vi "SeCrTs-AI SEQ MAIN.vi"(8 "error IO":errorcluster, 11 "Message Queue":refnum<queue>) -> (0 "error Out":errorcluster)   [LabVIEW 2022 SP3]
uses:
  <vilib>/Platform/TimedLoop/XDataNode/timing_clust.ctl
  <vilib>/Platform/TimedLoop/XDataNode/nitl_modes.ctl
  <vilib>/Platform/TimedLoop/XDataNode/wakeup.ctl
  RT Controls/SeCrTs-FGV Read write.ctl
  <vilib>/platform/TimedLoop/XDataNode/XDataNode.xnode
  <vilib>/Platform/TimedLoop/XDataNode/XDNodeRunTimeDep.lvlib
panel:
  out "array":string[](array[string])
  out "result":bool
  out "output array":string[](array[string])
  out "Failure case Seq":string[](array[string])
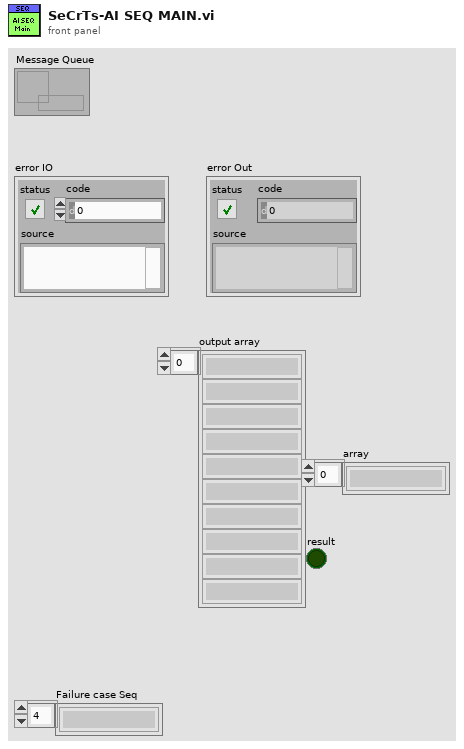
[diagram p1: front panel]
types:
  T1 = typedef "XDNodeRunTimeDep.lvlib/timing_clust.ctl" = cluster{"Expected End [f-1]":u64, "Actual End [f-1]":u64, "Finished Late? [f-1]":bool, "Expected End [i-1]":u64, "Actual End [i-1]":u64, "Finished Late? [i-1]":bool, "Expected Start [i]":u64, "Actual Start [i]":u64, "Expected Start [f]":u64, "Actual Start [f]":u64, "Source Name":string, "Structure Name":string, "Period":i64, "Deadline":i64, "Offset":i64, "Start":i64, "Priority":i32, "Timeout":i32, "Mode":T2, "Wakeup Reason":T3, "Error":errorcluster, "Source Type":string, "Secondary Source Type":string, "Global End Time":u64, "Global Start Time":u64, "Frame Duration":u64, "Iteration Duration":u64, "Assigned CPU":i32, "I/O Scan Engine Mode":u32}
  T2 = typedef "XDNodeRunTimeDep.lvlib/nitl_modes.ctl" = enum32{"No Change", "Process missed periods, maintain original phase", "Discard missed periods, maintain original phase", "Process missed periods, ignore original phase", "Discard missed periods, ignore original phase"}
  T3 = typedef "XDNodeRunTimeDep.lvlib/wakeup.ctl" = enum32{"Normal", "Aborted", "Asynchronous wakeup", "Timing source error", "Timed loop error", "Timeout"}
  T4 = typedef "SeCrTs-FGV Read write.ctl" = enum16{"Write", "Read"}
  T5 = cluster{"Manual HOLD":bool, "Automatic Hold AI":bool, "Abort":bool, "Automatic Hold DI":bool}
  T6 = cluster{"Start DAQ":bool, "Stop DAQ":bool, "RT Stop":bool, "RT Exit":bool, "Start Seq":bool}
  T7 = cluster{cluster{"Sr. No.":string, "Time CDT":string, "Component ID":string, "Data Type":string, "Condition":string, "Range/Position":string, "No of Samples for Pass":string, "Event Duration":string, "Continuous /Cumulative":string, "Expected Delay":string, "Failure case Seq":string, "Current Sequence":string}[]}[]
  T8 = cluster{"Sr. No.":string, "Time CDT":string, "Component ID":string, "Data Type":string, "Condition":string, "Range/Position":string, "No of Samples for Pass":string, "Event Duration":string, "Continuous /Cumulative":string, "Expected Delay":string, "Failure case Seq":string, "Current Sequence":string}[]
  T9 = cluster{"Sr. No.":string, "Time CDT":string, "Component ID":string, "Data Type":string, "Condition":string, "Range/Position":string, "No of Samples for Pass":string, "Event Duration":string, "Continuous /Cumulative":string, "Expected Delay":string, "Failure case Seq":string, "Current Sequence":string}
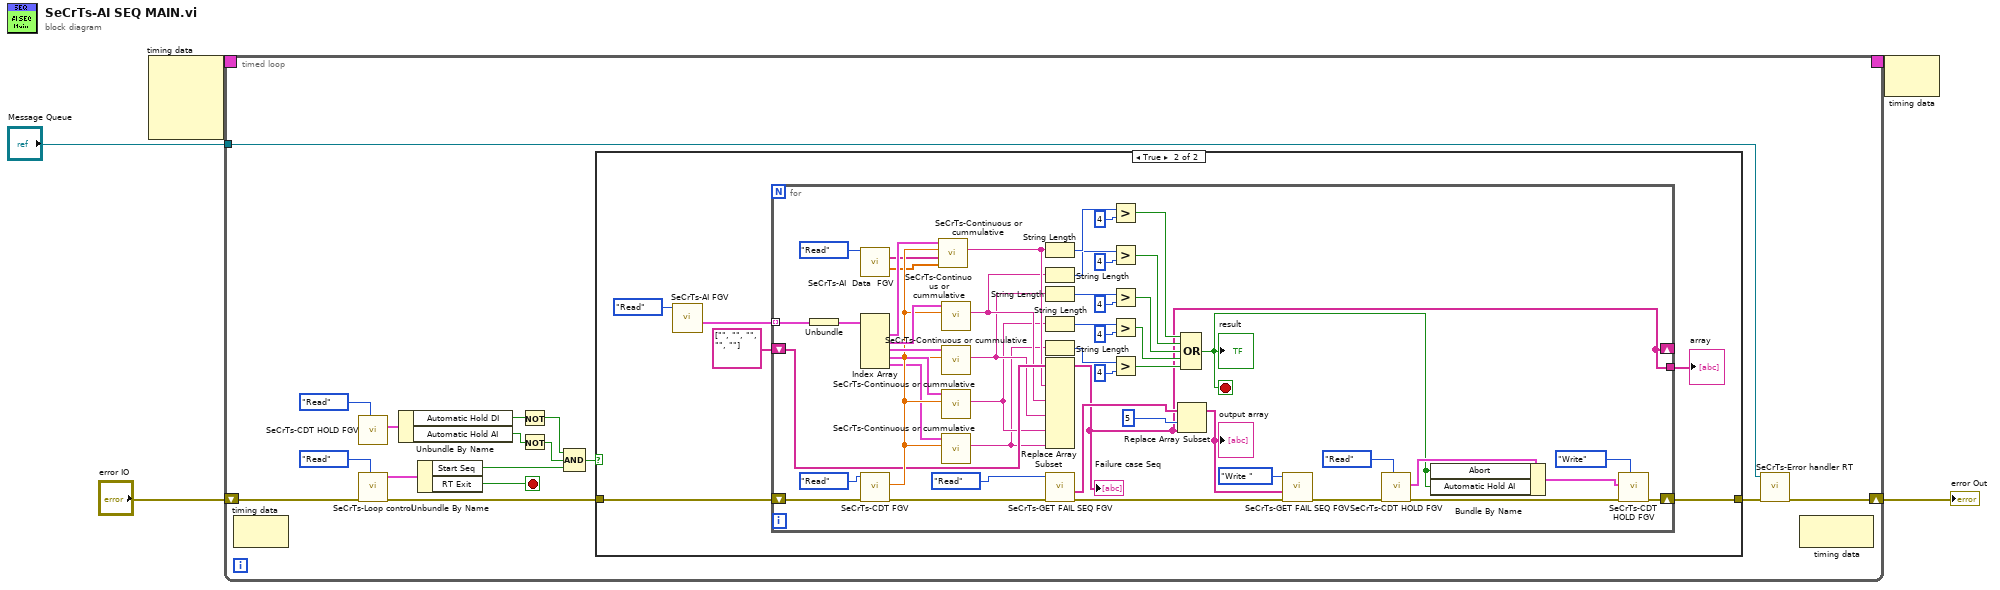
[diagram p0: block diagram]
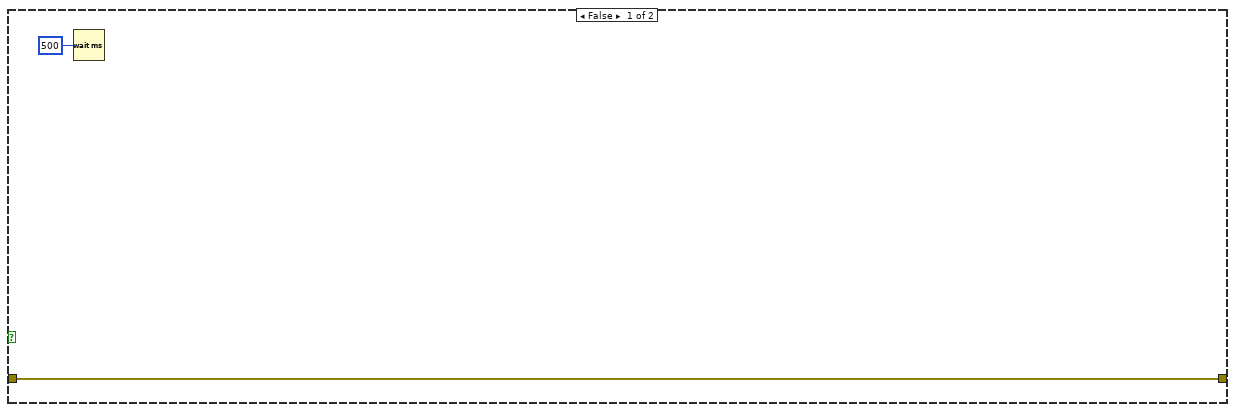
[diagram p2: hidden frame]
diagram:
  n1 = node-c288() -> (w3:T1)  [unwired: 4 in]
  n2 = timed-loop {
    timing: w3 -> [_]
    timing-out: [_] -> w2
    shift-right: [w15] -> w4
    shift-left: "error IO" -> [w11]
    tunnel: "Message Queue" -> [w6]
    stop <- w7 stop-if-true
    n3 = node-c288() -> ()  [unwired: 1 in, 1 out]
    n4 = call "SeCrTs-CDT HOLD FGV.vi"("Write/Read"=enum16{"Write", "Read"}."Read") -> ("HOLD and Abort Out"=w13:T5)  [unwired: 7 in, 1 out]
    n5 = call "SeCrTs-Loop control.vi"("Action"=enum16{"Init", "Write", "Read"}."Read", "error in (no error)"=w11) -> ("error Out"=w10:errorcluster, "Loop Control out"=w9:T6)  [unwired: 8 in]
    n6 = Unbundle By Name(w13) -> ("Automatic Hold DI"=w17:bool, "Automatic Hold AI"=w18:bool)
    n7 = Unbundle By Name(w9) -> ("Start Seq"=w8:bool, "RT Exit"=w7:bool)
    n8 = Not(x=w17) -> (.not. x?=w16:bool)
    n9 = Not(x=w18) -> (.not. x?=w20:bool)
    n10 = Compound Arithmetic op=AND(w16, w20, w8) -> (w19:bool)
    n11 = case shown="True" w19 {
      tunnel: w10 -> [w25 w31]
      tunnel: [w25 w26] -> w21
      frame False {
        n12 = Wait (ms)(milliseconds to wait=u32 500) -> ()  [unwired: 1 out]
      }
      frame True {
        n13 = call "SeCrTs-AI FGV.vi"("Enum"=enum16{"Read", "Write "}."Read") -> ("AI Seq  Out"=w28:T7)  [unwired: 9 in, 1 out]
        n14 = for {
          tunnel: w28 -> [w76] mode=indexing
          shift-right: [w38] -> w26
          shift-left: w31 -> [w74]
          shift-right: [w39] -> _
          shift-left: string[] ["", "", "", "", ""] ("array") -> [w72]
          tunnel: [w39] -> w27
          stop <- w32 stop-if-true
          n15 = Unbundle(w76) -> (w75:T8)
          n16 = call "SeCrTs-AI  Data  FGV.vi"("Write/Read"=SeCrTs-FGV_Read_write."Read") -> ("AI Channels Name LP"=w70:string[], "AI Y LP data"=w69:dbl[])  [unwired: 11 in, 2 out]
          n17 = Index Array(array=w75) -> (element #1=w80:T9, element #2=w79:T9, element #3=w78:T9, element #4=w77:T9, element #5=w66:T9)  [unwired: 5 in]
          n18 = call "SeCrTs-CDT FGV.vi"("error in (no error)"=w74, "Write/Read"=enum16{"Write", "Read"}."Read") -> ("error Out"=w65:errorcluster, "CDT Out"=w73:dbl)  [unwired: 8 in]
          n19 = call "SeCrTs-Continuous or cummulative.vi"("AI  data"=w69, "AI Channels Name LP"=w70, "CDT"=w73, "output cluster"=w80) -> ("Failure case Seq"=w63:string)  [unwired: 6 in, 1 out]
          n20 = call "SeCrTs-Continuous or cummulative.vi"("CDT"=w73, "output cluster"=w79) -> ("Failure case Seq"=w58:string)  [unwired: 8 in, 1 out]
          n21 = call "SeCrTs-Continuous or cummulative.vi"("CDT"=w73, "output cluster"=w78) -> ("Failure case Seq"=w51:string)  [unwired: 8 in, 1 out]
          n22 = call "SeCrTs-Continuous or cummulative.vi"("CDT"=w73, "output cluster"=w77) -> ("Failure case Seq"=w50:string)  [unwired: 8 in, 1 out]
          n23 = call "SeCrTs-Continuous or cummulative.vi"("CDT"=w73, "output cluster"=w66) -> ("Failure case Seq"=w48:string)  [unwired: 8 in, 1 out]
          n24 = String Length(string=w63) -> (length=w62:i32)
          n25 = String Length(string=w58) -> (length=w59:i32)
          n26 = String Length(string=w51) -> (length=w52:i32)
          n27 = String Length(string=w50) -> (length=w54:i32)
          n28 = String Length(string=w48) -> (length=w49:i32)
          n29 = Replace Array Subset(array=w72, new element #1=w63, new element #2=w58, new element #3=w51, new element #4=w50, new element #5=w48) -> (w39:string[])  [unwired: 5 in]
          "Failure case Seq" <- w39
          n30 = call "SeCrTs-GET FAIL SEQ FGV.vi"("error in"=w65, "Enum"=enum16{"Read", "Write "}."Read") -> ("error out"=w64:errorcluster, "Failure \ncase Seq"=w57:string[])  [unwired: 8 in]
          n31 = Greater?(x=w62, y=4) -> (0:w46:bool)
          n32 = Greater?(x=w59, y=4) -> (0:w45:bool)
          n33 = Greater?(x=w52, y=4) -> (0:w44:bool)
          n34 = Greater?(x=w54, y=4) -> (0:w43:bool)
          n35 = Greater?(x=w49, y=4) -> (0:w42:bool)
          n36 = Replace Array Subset(array=w57, new element=w39, index=5) -> (w55:string[])
          "output array" <- w55
          n37 = Compound Arithmetic op=OR(w46, w45, w44, w43, w42) -> (w32:bool)
          "result" <- w32
          n38 = call "SeCrTs-GET FAIL SEQ FGV.vi"("error in"=w64, "Failure \ncase Seq"=w55, "Enum"=enum16{"Read", "Write "}."Write ") -> ("error out"=w36:errorcluster)  [unwired: 7 in, 1 out]
          n39 = call "SeCrTs-CDT HOLD FGV.vi"("Write/Read"=enum16{"Write", "Read"}."Read", "error in (no error)"=w36) -> ("error Out"=w35:errorcluster, "HOLD and Abort Out"=w34:T5)  [unwired: 6 in]
          n40 = Bundle By Name(cluster=w34, "Abort"=w32, "Automatic Hold AI"=w32) -> (w33:T5)
          n41 = call "SeCrTs-CDT HOLD FGV.vi"("Write/Read"=enum16{"Write", "Read"}."Write", "error in (no error)"=w35, "HOLD and Abort"=w33) -> ("error Out"=w38:errorcluster)  [unwired: 5 in, 1 out]
        }
        "array" <- w27
      }
    }
    n42 = call "SeCrTs-Error handler RT.vi"("error in"=w21, "Message Queue"=w6) -> ("error out"=w15:errorcluster)  [unwired: 8 in, 1 out]
    n43 = node-c288() -> ()  [unwired: 1 in, 1 out]
  }
  "error Out" <- w4
  n44 = node-c288(w2) -> ()  [unwired: 1 out]
